vi "Auto Settings_MidSwitch_Scale.vi"(1 "Forward Ti me 1":dbl=1.0 min=0.0) -> ()   [LabVIEW 2017]
uses:
  <vilib>/Rock Robotics/Network Tables/NT Write Number.vi
panel:
  in  "Cube Shoot Speed 2":dbl=1.0 min=0.0
  in  "Cube Shoot Time 2":dbl=1.0 min=0.0
  in  "Cube Lift Speed 3":dbl=1.0 min=0.0
  in  "Cube Lift Time 3":dbl=1.0 min=0.0
  in  "Turn Speed 2":dbl=1.0 min=0.0
  in  "Turn Time 2":dbl=1.0 min=0.0
  in  "Forward Speed 5":dbl=1.0 min=0.0
  in  "Forward Time 5":dbl=1.0 min=0.0
  in  "CD Drive Speed":dbl=1.0 min=0.0
  in  "CD Drive Time":dbl=1.0 min=0.0
  in  "CD Wheel intake Speed":dbl=1.0 min=0.0
  in  "Turn Speed 1":dbl=1.0 min=0.0
  in  "Turn Time 1":dbl=1.0 min=0.0
  in  "Cube Lift Speed 2":dbl=1.0 min=0.0
  in  "Cube Lift Time 2":dbl=1.0 min=0.0
  in  "Forward Speed 4":dbl=1.0 min=0.0
  in  "Forward Time 4":dbl=1.0 min=0.0
  in  "Cube In Speed 1":dbl=1.0 min=0.0
  in  "Cube In Time 1":dbl=1.0 min=0.0
  in  "Forward Speed 3":dbl=1.0 min=0.0
  in  "Forward Time 3":dbl=1.0 min=0.0
  in  "Cube Lift Speed 1":dbl=1.0 min=0.0
  in  "Cube Lift Time 1":dbl=1.0 min=0.0
  in  "Strafe Speed 2":dbl=1.0 min=0.0
  in  "Strafe Ti me 2":dbl=1.0 min=0.0
  in  "Forward Speed 2":dbl=1.0 min=0.0
  in  "Forward Time 2":dbl=1.0 min=0.0
  in  "Strafe Speed 1":dbl=1.0 min=0.0
  in  "Strafe Ti me 1":dbl=1.0 min=0.0
  in  "Forward Speed 1":dbl=1.0 min=0.0
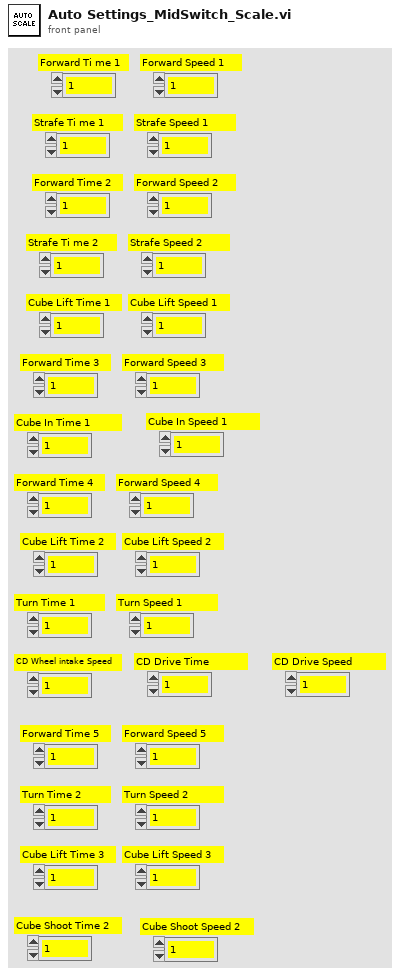
[diagram p1: front panel]
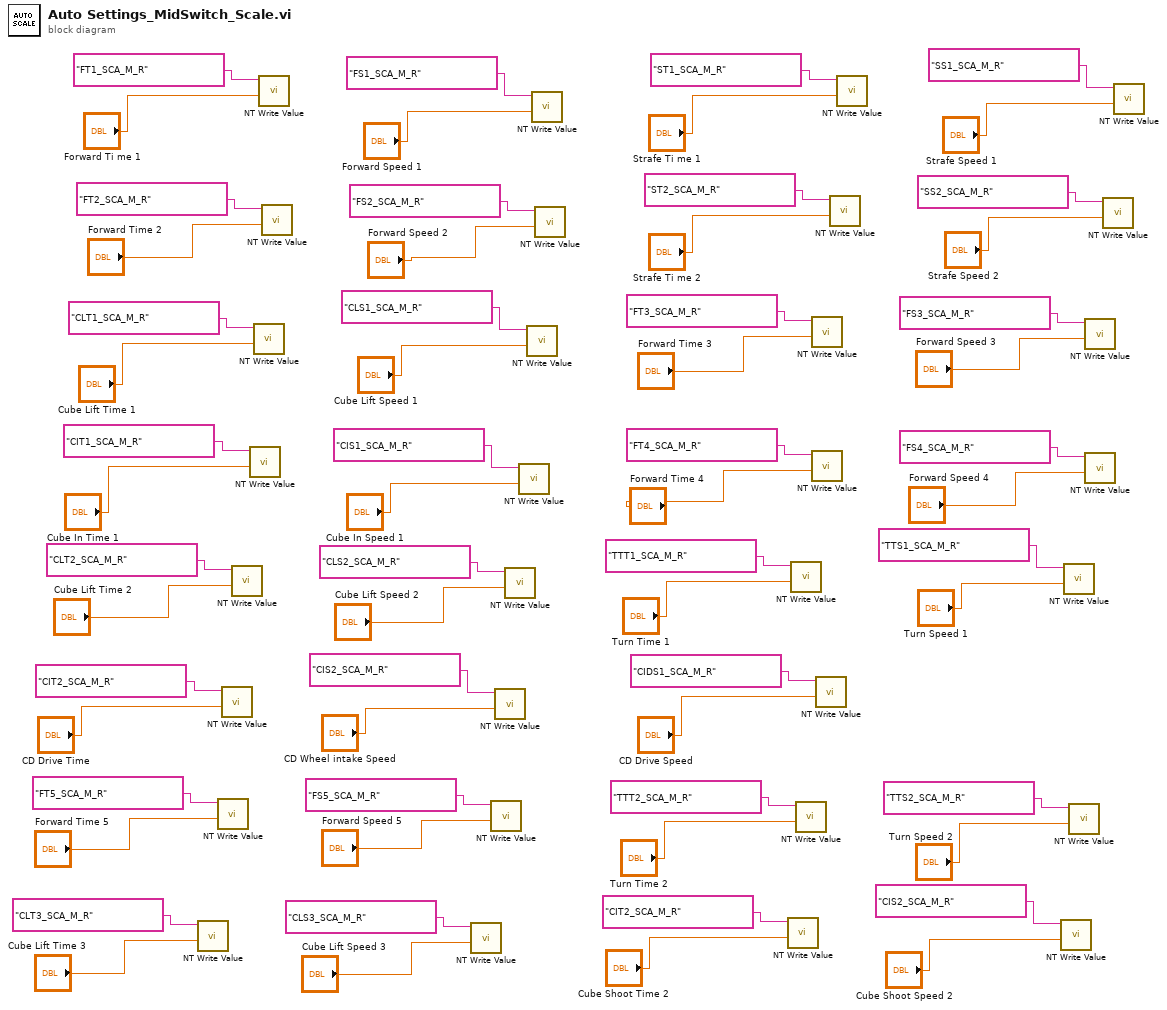
[diagram p0: block diagram]
diagram:
  n1 = call-poly <vilib>:"NT Write Value.vi"("Numeric"="Cube Lift Time 3", "Name"="CLT3_SCA_M_R") -> ()  [unwired: 9 in, 1 out]
  n2 = call-poly <vilib>:"NT Write Value.vi"("Numeric"="Forward Time 5", "Name"="FT5_SCA_M_R") -> ()  [unwired: 9 in, 1 out]
  n3 = call-poly <vilib>:"NT Write Value.vi"("Numeric"="CD Drive Time", "Name"="CIT2_SCA_M_R") -> ()  [unwired: 9 in, 1 out]
  n4 = call-poly <vilib>:"NT Write Value.vi"("Numeric"="Cube Lift Time 2", "Name"="CLT2_SCA_M_R") -> ()  [unwired: 9 in, 1 out]
  n5 = call-poly <vilib>:"NT Write Value.vi"("Numeric"="Cube In Time 1", "Name"="CIT1_SCA_M_R") -> ()  [unwired: 9 in, 1 out]
  n6 = call-poly <vilib>:"NT Write Value.vi"("Numeric"="Cube Lift Time 1", "Name"="CLT1_SCA_M_R") -> ()  [unwired: 9 in, 1 out]
  n7 = call-poly <vilib>:"NT Write Value.vi"("Numeric"="Forward Ti me 1", "Name"="FT1_SCA_M_R") -> ()  [unwired: 9 in, 1 out]
  n8 = call-poly <vilib>:"NT Write Value.vi"("Numeric"="Forward Time 2", "Name"="FT2_SCA_M_R") -> ()  [unwired: 9 in, 1 out]
  n9 = call-poly <vilib>:"NT Write Value.vi"("Numeric"="Cube Lift Speed 3", "Name"="CLS3_SCA_M_R") -> ()  [unwired: 9 in, 1 out]
  n10 = call-poly <vilib>:"NT Write Value.vi"("Numeric"="Forward Speed 5", "Name"="FS5_SCA_M_R") -> ()  [unwired: 9 in, 1 out]
  n11 = call-poly <vilib>:"NT Write Value.vi"("Numeric"="CD Wheel intake Speed", "Name"="CIS2_SCA_M_R") -> ()  [unwired: 9 in, 1 out]
  n12 = call-poly <vilib>:"NT Write Value.vi"("Numeric"="Cube Lift Speed 2", "Name"="CLS2_SCA_M_R") -> ()  [unwired: 9 in, 1 out]
  n13 = call-poly <vilib>:"NT Write Value.vi"("Numeric"="Cube In Speed 1", "Name"="CIS1_SCA_M_R") -> ()  [unwired: 9 in, 1 out]
  n14 = call-poly <vilib>:"NT Write Value.vi"("Numeric"="Cube Lift Speed 1", "Name"="CLS1_SCA_M_R") -> ()  [unwired: 9 in, 1 out]
  n15 = call-poly <vilib>:"NT Write Value.vi"("Numeric"="Forward Speed 1", "Name"="FS1_SCA_M_R") -> ()  [unwired: 9 in, 1 out]
  n16 = call-poly <vilib>:"NT Write Value.vi"("Numeric"="Forward Speed 2", "Name"="FS2_SCA_M_R") -> ()  [unwired: 9 in, 1 out]
  n17 = call-poly <vilib>:"NT Write Value.vi"("Numeric"="Cube Shoot Time 2", "Name"="CIT2_SCA_M_R") -> ()  [unwired: 9 in, 1 out]
  n18 = call-poly <vilib>:"NT Write Value.vi"("Numeric"="Turn Time 1", "Name"="TTT1_SCA_M_R") -> ()  [unwired: 9 in, 1 out]
  n19 = call-poly <vilib>:"NT Write Value.vi"("Numeric"="Turn Time 2", "Name"="TTT2_SCA_M_R") -> ()  [unwired: 9 in, 1 out]
  n20 = call-poly <vilib>:"NT Write Value.vi"("Numeric"="Forward Time 3", "Name"="FT3_SCA_M_R") -> ()  [unwired: 9 in, 1 out]
  n21 = call-poly <vilib>:"NT Write Value.vi"("Numeric"="Forward Time 4", "Name"="FT4_SCA_M_R") -> ()  [unwired: 9 in, 1 out]
  n22 = call-poly <vilib>:"NT Write Value.vi"("Numeric"="CD Drive Speed", "Name"="CIDS1_SCA_M_R") -> ()  [unwired: 9 in, 1 out]
  n23 = call-poly <vilib>:"NT Write Value.vi"("Numeric"="Strafe Ti me 2", "Name"="ST2_SCA_M_R") -> ()  [unwired: 9 in, 1 out]
  n24 = call-poly <vilib>:"NT Write Value.vi"("Numeric"="Strafe Ti me 1", "Name"="ST1_SCA_M_R") -> ()  [unwired: 9 in, 1 out]
  n25 = call-poly <vilib>:"NT Write Value.vi"("Numeric"="Cube Shoot Speed 2", "Name"="CIS2_SCA_M_R") -> ()  [unwired: 9 in, 1 out]
  n26 = call-poly <vilib>:"NT Write Value.vi"("Numeric"="Turn Speed 1", "Name"="TTS1_SCA_M_R") -> ()  [unwired: 9 in, 1 out]
  n27 = call-poly <vilib>:"NT Write Value.vi"("Numeric"="Turn Speed 2", "Name"="TTS2_SCA_M_R") -> ()  [unwired: 9 in, 1 out]
  n28 = call-poly <vilib>:"NT Write Value.vi"("Numeric"="Forward Speed 3", "Name"="FS3_SCA_M_R") -> ()  [unwired: 9 in, 1 out]
  n29 = call-poly <vilib>:"NT Write Value.vi"("Numeric"="Forward Speed 4", "Name"="FS4_SCA_M_R") -> ()  [unwired: 9 in, 1 out]
  n30 = call-poly <vilib>:"NT Write Value.vi"("Numeric"="Strafe Speed 2", "Name"="SS2_SCA_M_R") -> ()  [unwired: 9 in, 1 out]
  n31 = call-poly <vilib>:"NT Write Value.vi"("Numeric"="Strafe Speed 1", "Name"="SS1_SCA_M_R") -> ()  [unwired: 9 in, 1 out]
